vi "CCD_Exposure_2-D v.82.vi"(7 "CCD GPIB Address":u16=1, 8 "error in":errorcluster, 10 "Shutter Enabled":bool=TRUE, 11 "Exposuretime (s)":dbl=0.5 format="%.2f") -> (0 "Error Out":errorcluster, 1 "#PixelOverflow":u32, 2 "PixelOverflow":bool, 3 "The Data":i32[][](array[numeric])=[[1198, 1190, 1193, 1194, 1189, 1188, 1196, 1190, 1202, 1191, 1193, 1192, 1199, 1189, 1194, 1189, 1197, 1191, 1187, 1192, 1195, 1189, 1195, 1191, 1199, 1194, 1192, 1191, 1193, 1197, 1193, 1193, 1194, 1200, 1191, 1190, 1187, 1195, 1189, 1188, 1191, 1194, 1187, 1192, 1198, 1193, 1190, 1192, 1190, 1193, 1191, 1190, 1191, 1189, 1192, 1194, 1190, 1193, 1193, 1191, 1194, 1182, 1190, 1188, 1199, 1192, 1196, 1195, 1186, 1189, 1188, 1185, 1194, 1187, 1193, 1194, 1190, 1189, 1189, 1187, 1196, 1195, 1191, 1197, 1192, 1200, 1187, 1194, 1189, 1193, 1195, 1196, 1186, 1192, 1190, 1194, 1194, 1190, 1191, 1193, 1197, 1197, 1185, 1199, 1190, 1195, 1196, 1184, 1193, 1193, 1193, 1191, 1189, 1190, 1199, 1193, 1191, 1194, 1191, 1192, 1186, 1190, 1194, 1189, 1194, 1190, 1191, 1192, 1192, 1196, 1192, 1192, 1189, 1193, 1198, 1186, 1191, 1193, 1187, 1194, 1190, 1190, 1191, 1189, 1194, 1195, 1189, 1192, 1185, 1193, 1192, 1192, 1189, 1191, 1191, 1190, 1196, 1194, 1193, 1191, 1189, 1191, 1196, 1192, 1192, 1189, 1196, 1191, 1193, 1192, 1188, 1190, 1194, 1192, 1185, 1191, 1194, 1191, 1189, 1195, 1192, 1196, 1190, 1193, 1191, 1189, 1194, 1195, 1191, 1187, 1190, 1196, 1196, 1192, 1197, 1191, 1189, 1192, 1192, 1200, 1192, 1193, 1190, 1192, 1187, 1198, 1186, 1196, 1201, 1199, 1200, 1191, 1196, 1200, 1192, 1191, 1193, 1185, 1192, 1194, 1186, 1190, 1188, 1189, 1201, 1197, 1191, 1194, 1193, 1194, 1195, 1198, 1200, 1192, 1192, 1193, 1193, 1195, 1187, 1193, 1192, 1187, 1189, 1186, 1191, 1197, 1191, 1200, 1194, 1192, 1187, 1196, 1191, 1191, 1196, 1187, 1190, 1193, 1189, 1193, 1190, 1188, 1188, 1190, 1197, 1188, 1191, 1195, 1188, 1191, 1188, 1194, 1193, 1187, 1200, 1192, 1197, 1190, 1196, 1200, 1191, 1189, 1193, 1189, 1186, 1196, 1185, 1198, 1195, 1186, 1191, 1197, 1191, 1193, 1195, 1193, 1191, 1198, 1189, 1183, 1200, 1197, 1192, 1192, 1192, 1196, 1191, 1190, 1194, 1188, 1198, 1193, 1195, 1190, 1187, 1192, 1191, 1195, 1188, 1190, 1191, 1187, 1189, 1185, 1189, 1196, 1198, 1191, 1190, 1196, 1197, 1193, 1187, 1186, 1195, 1191, 1193, 1192, 1196, 1190, 1192, 1192, 1192, 1190, 1195, 1192, 1191, 1193, 1197, 1184, 1190, 1188, 1192, 1194, 1190, 1193, 1195, 1195, 1194, 1189, 1193, 1191, 1194, 1186, 1189, 1192, 1191, 1182, 1190, 1197, 1194, 1188, 1193, 1191, 1186, 1194, 1197, 1193, 1191, 1187, 1194, 1194, 1191, 1189, 1195, 1194, 1189, 1196, 1187, 1186, 1192, 1194, 1196, 1191, 1193, 1191, 1188, 1190, 1199, 1198, 1196, 1196, 1190, 1194, 1191, 1194, 1187, 1195, 1190, 1194, 1196, 1194, 1189, 1193, 1189, 1194, 1189, 1195, 1192, 1194, 1193, 1191, 1197, 1187, 1189, 1189, 1188, 1197, 1192, 1189, 1193, 1194, 1183, 1202, 1187, 1192, 1184, 1188, 1186, 1193, 1189, 1195, 1189, 1193, 1197, 1189, 1194, 1191, 1194, 1192, 1191, 1191, 1196, 1194, 1190, 1193, 1192, 1195, 1197, 1198, 1193, 1202, 1196, 1194, 1194, 1190, 1193, 1190, 1195, 1192, 1187, 1194, 1197, 1190, 1194, 1189, 1198, 1192, 1191, 1192, 1192, 1191, 1191, 1193, 1191, 1191, 1198, 1186, 1192, 1185, 1185, 1188, 1194, 1196, 1194, 1195, 1190, 1194, 1191, 1190, 1195, 1191, 1191, 1195, 1192, 1194, 1201, 1187, 1191, 1195, 1187, 1192, 1192, 1193, 1200, 1188, 1189, 1189, 1197, 1189, 1188, 1197, 1195, 1191, 1189, 1190, 1195, 1189, 1191, 1194, 1186, 1192, 1190, 1191, 1188, 1195, 1192, 1191, 1191, 1199, 1190, 1190, 1190, 1192, 1187, 1193, 1197, 1197, 1186, 1193, 1189, 1192, 1197, 1184, 1187, 1188, 1192, 1192, 1192, 1189, 1192, 1190, 1194, 1191, 1186, 1196, 1194, 1189, 1193, 1191, 1186, 1189, 1193, 1195, 1196, 1197, 1199, 1194, 1190, 1193, 1194, 1190, 1198, 1196, 1194, 1195, 1194, 1184, 1188, 1195, 1197, 1190, 1194, 1190, 1191, 1195, 1198, 1188, 1193, 1194, 1195, 1198, 1195, 1191, 1197, 1192, 1198, 1190, 1196, 1191, 1194, 1188, 1189, 1198, 1192, 1198, 1195, 1185, 1191, 1193, 1192, 1197, 1195, 1195, 1195, 1193, 1190, 1190, 1190, 1198, 1195, 1191, 1194, 1190, 1190, 1194, 1194, 1195, 1192, 1190, 1194, 1195, 1192, 1192, 1194, 1189, 1192, 1193, 1188, 1194, 1195, 1196, 1193, 1192, 1201, 1191, 1198, 1197, 1191, 1192, 1191, 1194, 1193, 1188, 1192, 1189, 1183, 1189, 1190, 1192, 1189, 1196, 1193, 1197, 1185, 1193, 1189, 1191, 1196, 1195, 1193, 1193, 1191, 1189, 1193, 1192, 1192, 1192, 1190, 1191, 1193, 1193, 1197, 1195, 1189, 1193, 1188, 1194, 1197, 1194, 1195, 1196, 1190, 1194, 1188, 1197, 1195, 1191, 1195, 1192, 1194, 1188, 1190, 1197, 1197, 1191, 1187, 1197, 1191, 1193, 1188, 1191, 1194, 1193, 1195, 1192, 1195, 1189, 1193, 1193, 1195, 1190, 1192, 1196, 1188, 1187, 1193, 1192, 1192, 1194, 1185, 1199, 1190, 1193, 1191, 1198, 1189, 1190, 1191, 1190, 1193, 1195, 1186, 1190, 1193, 1191, 1189, 1197, 1193, 1198, 1190, 1192, 1193, 1191, 1196, 1193, 1196, 1190, 1190, 1198, 1192, 1199, 1198, 1190, 1191, 1191, 1196, 1190, 1196, 1195, 1191, 1196, 1195, 1193, 1190, 1190, 1195, 1193, 1187, 1197, 1185, 1191, 1189, 1191, 1193, 1192, 1188, 1196, 1193, 1191, 1193, 1193, 1190, 1192, 1192, 1192, 1195, 1191, 1195, 1189, 1189, 1191, 1191, 1185, 1192, 1191, 1193, 1201, 1199, 1197, 1206, 1201, 1207, 1200, 1198, 1195, 1188, 1194, 1186, 1190, 1197, 1188, 1193, 1196, 1193, 1192, 1192, 1188, 1196, 1186, 1193, 1194, 1188, 1190, 1190, 1192, 1190, 1191, 1191, 1200, 1192, 1199, 1193, 1190, 1190, 1199, 1187, 1193, 1190, 1188, 1194, 1194, 1196, 1194, 1195, 1190, 1187, 1187, 1196, 1193, 1199, 1190, 1193, 1193, 1191, 1198, 1192, 1193, 1192, 1193, 1189, 1189, 1197, 1189, 1194, 1193, 1192, 1185, 1198, 1193, 1189, 1192, 1193, 1196, 1190, 1195, 1189, 1196, 1198, 1190, 1191, 1193, 1186, 1189, 1195, 1188, 1197, 1188, 1191, 1185, 1190, 1193, 1188, 1198, 1192, 1193, 1194, 1194, 1189, 1184, 1193, 1199, 1193, 1192, 1193, 1190, 1196, 1191, 1192, 1189, 1194, 1188, 1189, 1190, 1190, 1192, 1195, 1188, 1190, 1192, 1189, 1197, 1192, 1194, 1187, 1196, 1192, 1194, 1185, 1187, 1187, 1191, 1195, 1190, 1186, 1183, 1194, 1194, 1192, 1192, 1188, 1193, 1195, 1189, 1190, 1191, 1192, 1196, 1186, 1195, 1191, 1185, 1191, 1187, 1190, 1188, 1189, 1187, 1196, 1191, 1190, 1191, 1190, 1196, 1195, 1186, 1187, 1187, 1188, 1194, 1192, 1192, 1192, 1189, 1192, 1191, 1188, 1188, 1187, 1187, 1190, 1186, 1191, 1195, 1192, 1196, 1193, 1192, 1191, 1189, 1187, 1193, 1188, 1189, 1194, 1191, 1185, 1193, 1191, 1196, 1196, 1199, 1195, 1211]], 4 "GPIB Status":i16=-1, 5 "sd":i32=1024, 6 "Setup String":string="ldu,0,256,16;sdu,0,1024,1024;cl0;omrm;sron")   [LabVIEW 2021]
doc: "Get the 2-D CCD data. The CCD GPIB address is more or less fixed.\nThe setup string uses global variable."
uses:
  Globals and TypeDefs/Global Varibal Control.vi
panel:
  out "Data Dimensions":i32[](array[numeric])
  out "read status":bool[](array[boolean])
  out "\"TS\" status":bool[](array[boolean])
  out "\"ST\" status":bool[](array[boolean])
  out "RQS  poll response":i16
  out "InitialArray Length":i32=16384
  out "ld":i32=16
  out "Array Length":i32=1024
  # "8: ON=complete;         13: ON=EOI detected"
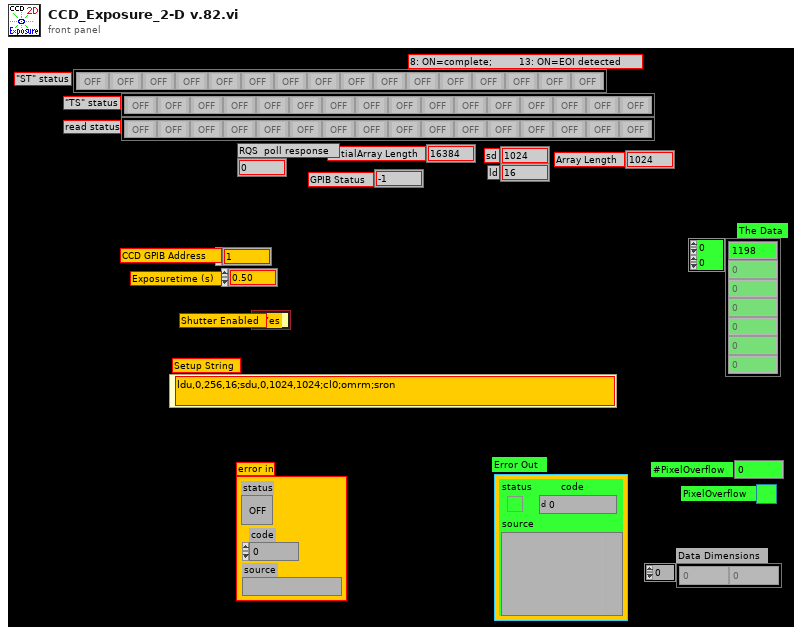
[diagram p1: front panel]
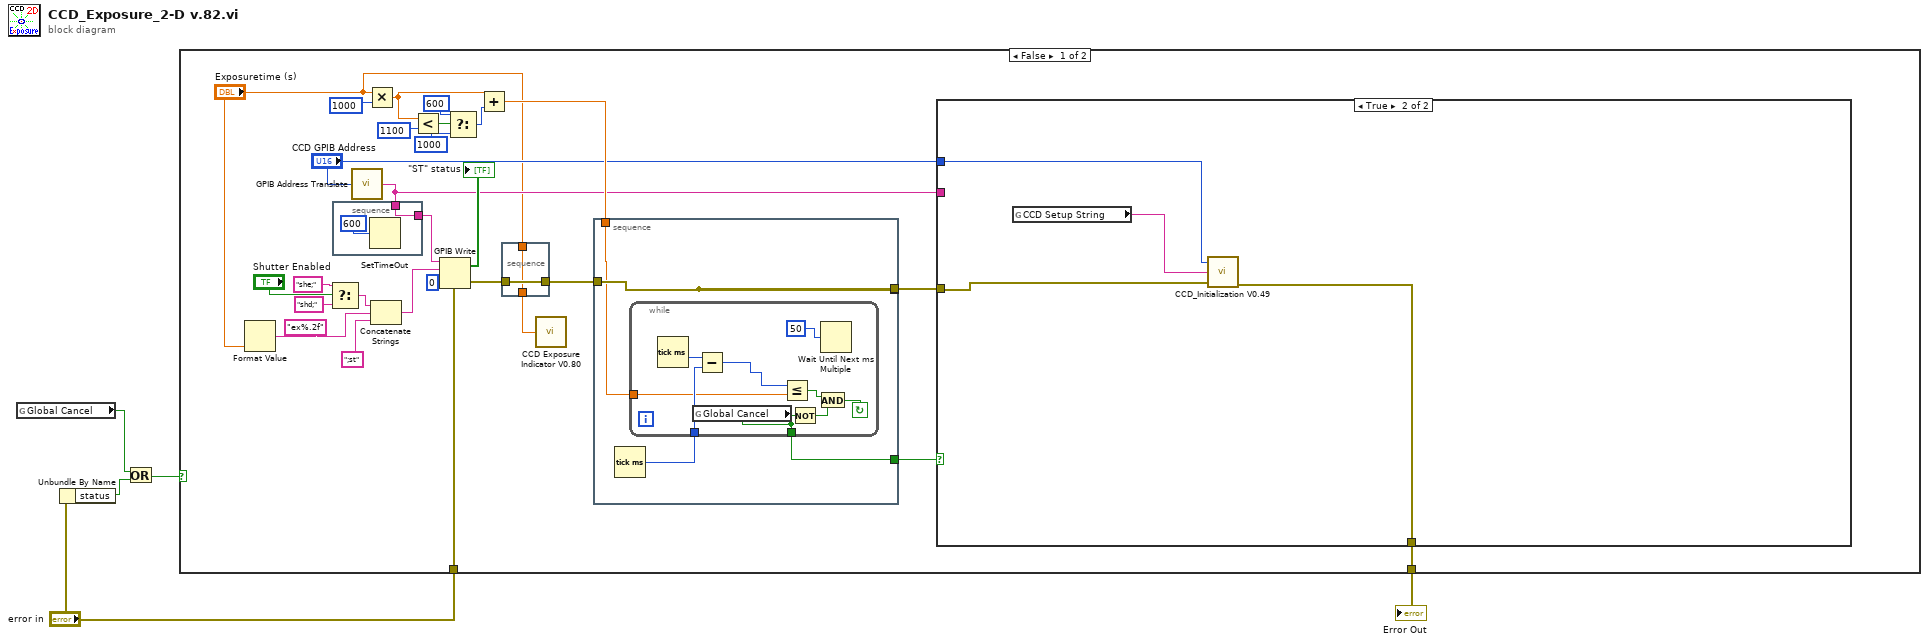
[diagram p0: block diagram]
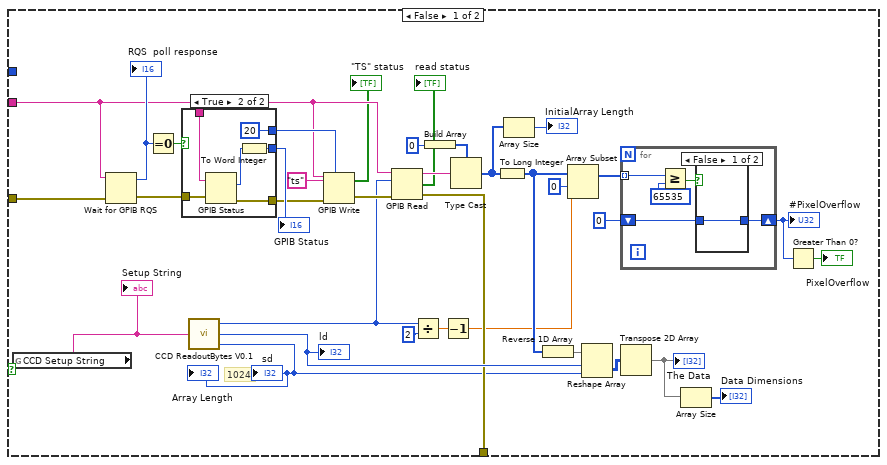
[diagram p2: hidden frame]
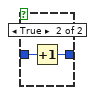
[diagram p3: hidden frame]
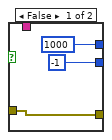
[diagram p4: hidden frame]
diagram:
  n1 = global read "Global Varibal Control.vi" "Global Cancel"() -> (w1:bool)
  n2 = Unbundle By Name("error in") -> ("status"=w4:bool)
  n3 = Or(x=w1, y=w4) -> (x .or. y?=w2:bool)
  n4 = case shown="False" w2 {
    tunnel: [w26 w108] -> w5
    tunnel: "error in" -> [w21 w108]
    frame False {
      n5 = Format Value(format string="ex%.2f", value (0)="Exposuretime (s)") -> (output string=w13:string)  [unwired: 1 in]
      n6 = Select(t="she;", s="Shutter Enabled", f="shd;") -> (s? t:f=w14:string)
      n7 = call "GPIB Address Translate.vi"("GPIB Address"="CCD GPIB Address") -> ("GPIB Address String"=w19:string)
      n8 = stacked-sequence {
        tunnel: [w106] -> w25
        tunnel: w19 -> [w106]
        frame #0 {
          n9 = SetTimeOut(1:600) -> ()  [unwired: 1 out]
        }
      }
      n10 = Multiply(x="Exposuretime (s)", y=1000) -> (x*y=w30:dbl)
      n11 = Concatenate Strings(w14, w13, ";st") -> (w12:string)
      n12 = Less?(x=w30, y=1100) -> (x < y?=w32:bool)
      n13 = GPIB Write(0:w25, 1:w12, 2:i16 0 ("mode (0)"), 3:w21) -> (5:→"\"ST\" status":bool[], 6:w10:errorcluster)  [unwired: 1 in]
      n14 = Select(t=u32 600, s=w32, f=u32 1000 ("Added are a minimum of 600ms")) -> (s? t:f=w29:u32)
      n15 = Add(x=w30, y=w29) -> (x+y=w28:dbl)
      n16 = stacked-sequence {
        tunnel: [w92] -> w9
        tunnel: w10 -> [w92]
        tunnel: [w91] -> w7
        tunnel: "Exposuretime (s)" -> [w91]
        frame #0 {
        }
      }
      n17 = call "CCD Exposure Indicator V0.80.vi"("ExpTime"=w7) -> ()  [unwired: 4 in]
      n18 = stacked-sequence {
        tunnel: w28 -> [w95]
        tunnel: w9 -> [w96]
        tunnel: [w96] -> _
        tunnel: [w96] -> w23
        tunnel: [w93] -> w6
        frame #0 {
          n19 = Tick Count (ms)() -> (millisecond timer value=w94:u32)
          n20 = while {
            tunnel: [w97] -> w93
            tunnel: w95 -> [w102]
            tunnel: w94 -> [w104]
            stop <- w99 continue-if-true
            n21 = Tick Count (ms)() -> (millisecond timer value=w105:u32)
            n22 = global read "Global Varibal Control.vi" "Global Cancel"() -> (w97:bool)
            n23 = Subtract(x=w105, y=w104) -> (x-y=w98:u32)
            n24 = Less Or Equal?(x=w98, y=w102) -> (x <= y?=w100:bool)
            n25 = Not(x=w97) -> (.not. x?=w101:bool)
            n26 = And(x=w100, y=w101) -> (x .and. y?=w99:bool)
            n27 = Wait Until Next ms Multiple(millisecond multiple=u32 50) -> ()  [unwired: 1 out]
          }
        }
      }
      n28 = case shown="True" w6 {
        tunnel: [w59 w89] -> w26
        tunnel: w23 -> [w58 w90]
        tunnel: w19 -> [w47 _]
        tunnel: "CCD GPIB Address" -> [_ w88]
        frame False {
          # "1024"
          n29 = global read "Global Varibal Control.vi" "CCD Setup String"() -> (w35:string)
          "Setup String" <- w35
          n30 = Wait for GPIB RQS(2:w58, 4:w47) -> (0:w46:errorcluster, 1:w57:i16)  [unwired: 1 in]
          "RQS  poll response" <- w57
          n31 = Equal To 0?(x=w57) -> (x = 0?=w56:bool)
          n32 = case shown="True" w56 {
            tunnel: w47 -> [_ w86]
            tunnel: [i16 -1 w85] -> w55
            tunnel: [u32 1000 u32 20] -> w53
            tunnel: w46 -> [w78 w82]
            tunnel: [w78 w81] -> w45
            frame False {
            }
            frame True {
              n33 = GPIB Status(0:w86, 1:w82) -> (3:w84:i16, 5:w81:errorcluster)  [unwired: 2 out]
              n34 = To Word Integer(number=w84) -> (16bit integer=w85:i16)
            }
          }
          "GPIB Status" <- w55
          n35 = call "CCD ReadoutBytes V0.1.vi"("CCD Setup String"=w35) -> ("Bytes for Readout"=w51:i32, "LD Bytes"=w63:i32, "SD Bytes"=w38:i32)
          "Array Length" <- w38
          "sd" <- w38
          "ld" <- w63
          n36 = GPIB Write(0:w47, 1:"ts" ("String to Write"), 3:w45, 4:w53) -> (5:→"\"TS\" status":bool[], 6:w52:errorcluster)  [unwired: 1 in]
          n37 = GPIB Read(0:w47, 1:w51, 3:w52) -> (5:w62:string, 6:→"read status":bool[], 7:w59:errorcluster)  [unwired: 2 in]
          n38 = Divide(x=w51, y=2) -> (x/y=w49:dbl)
          n39 = Build Array(u16 0) -> (w67:u16[])
          n40 = Decrement(x=w49) -> (x-1=w48:dbl)
          n41 = Type Cast(type=w67, x=w62) -> (*(type *) &x=w69:u16[])
          n42 = To Long Integer(number=w69) -> (32bit integer=w60:i32[])
          n43 = Array Size(array=w69) -> (size(s)=→"InitialArray Length":i32)
          n44 = Reverse 1D Array(array=w60) -> (reversed array=w64:i32[])
          n45 = Array Subset(array=w60, index=0, length=w48) -> (w42:i32[])
          n46 = Reshape Array(w64, w63, w38) -> (w65:i32[][])
          n47 = for {
            tunnel: w42 -> [w73] mode=indexing
            shift-right: [w71] -> w40
            shift-left: u32 0 -> [w70]
            n48 = Greater Or Equal?(x=w73, y=65535) -> (x >= y?=w72:bool)
            n49 = case shown="False" w72 {
              tunnel: [w75 w77] -> w71
              tunnel: w70 -> [w75 w76]
              frame False {
              }
              frame True {
                n50 = Increment(x=w76) -> (x+1=w77:u32)
              }
            }
          }
          "#PixelOverflow" <- w40
          n51 = Transpose 2D Array(2D array=w65) -> (transposed array=w37:i32[][])
          "The Data" <- w37
          n52 = Array Size(array=w37) -> (size(s)=→"Data Dimensions":i32[])
          n53 = Greater Than 0?(x=w40) -> (x > 0?=→"PixelOverflow":bool)
        }
        frame True {
          n54 = global read "Global Varibal Control.vi" "CCD Setup String"() -> (w87:string)
          n55 = call "CCD_Initialization V0.49.vi"("error in"=w90, "Setup String"=w87, "CCD GPIB Address"=w88) -> ("error out"=w89:errorcluster)  [unwired: 2 in, 3 out]
        }
      }
    }
    frame True {
    }
  }
  "Error Out" <- w5
